vi "Start Trigger Date.vi"(8 "error in (no error)":errorcluster, 10 "Start date":timestamp, 11 "VISA resource name":refnum<visa-resource-name>) -> (0 "error out":errorcluster, 3 "VISA resource name out":refnum<visa-resource-name>)   [LabVIEW 2017, in "Sefram DAS220.lvlib"]
doc: "Set start trigger in date mode : wait for a date to start recording."
uses:
  <instrlib>/Sefram DAS220/Sefram DAS220.lvlib
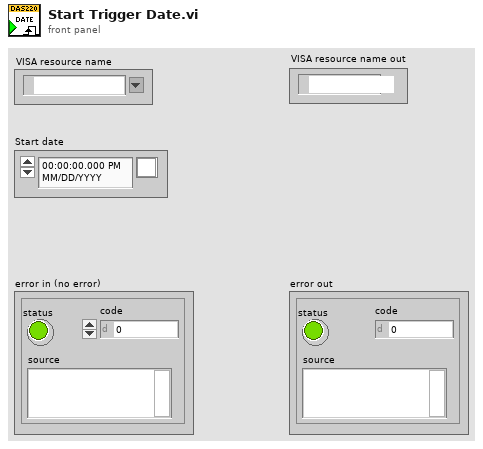
[diagram p1: front panel]
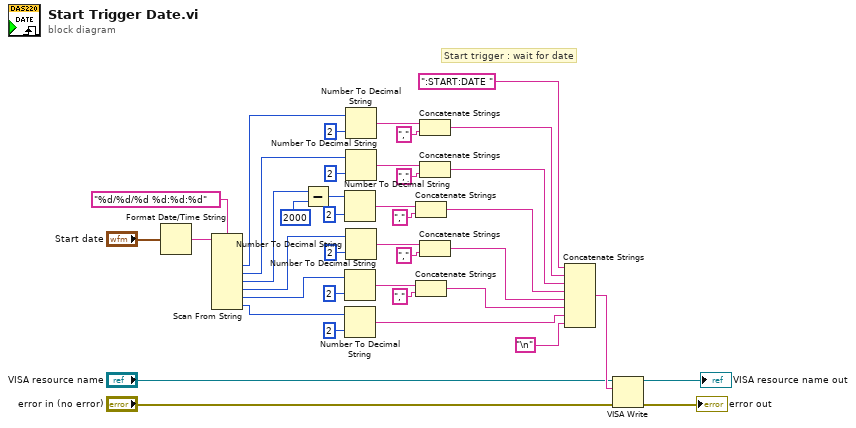
[diagram p0: block diagram]
diagram:
  # "Start trigger : wait for date"
  n1 = Format Date/Time String(seconds (now)="Start date") -> (date/time string=w30:string)  [unwired: 2 in]
  n2 = Scan From String(format string="%d/%d/%d %d:%d:%d", input string=w30) -> (output 1=w20:i32, output 2=w19:i32, output 3=w15:i32, output 4=w18:i32, output 5=w17:i32, output 6=w16:i32)  [unwired: 8 in, 3 out]
  n3 = Subtract(x=w15, y=2000) -> (x-y=w13:i32)
  n4 = Number To Decimal String(number=w13, width (-)=i16 2) -> (decimal integer string=w25:string)
  n5 = Number To Decimal String(number=w17, width (-)=i16 2) -> (decimal integer string=w33:string)
  n6 = Number To Decimal String(number=w16, width (-)=i16 2) -> (decimal integer string=w6:string)
  n7 = Number To Decimal String(number=w20, width (-)=i16 2) -> (decimal integer string=w22:string)
  n8 = Number To Decimal String(number=w19, width (-)=i16 2) -> (decimal integer string=w27:string)
  n9 = Number To Decimal String(number=w18, width (-)=i16 2) -> (decimal integer string=w35:string)
  n10 = Concatenate Strings(w25, "," ("string")) -> (w9:string)
  n11 = Concatenate Strings(w33, "," ("string")) -> (w7:string)
  n12 = Concatenate Strings(w22, "," ("string")) -> (w11:string)
  n13 = Concatenate Strings(w27, "," ("string")) -> (w10:string)
  n14 = Concatenate Strings(w35, "," ("string")) -> (w8:string)
  n15 = Concatenate Strings(":START:DATE " ("string"), w11, w10, w9, w8, w7, w6, "\n") -> (w40:string)
  n16 = VISA Write(VISA resource name="VISA resource name", write buffer=w40, error in (no error)="error in (no error)") -> (VISA resource name out=→"VISA resource name out":refnum<visa-resource-name>, error out=→"error out":errorcluster)  [unwired: 1 out]
